vi "Pod Health Status Simulator.vi"(10 "Simulated Telemetry":T1={"Friction Brake (mA)"=300.0, "Mag Brake (mA)"=306.4516129032258, "Prim. Batt. (V)"=11.822168912654636, "Backup Batt. (V)"=11.62716511535498, "High Pressure (PSI)"=2438.59649122807, "Med. Pressure (PSI)"=254.3859649122807, "Low Pressure (PSI)"=50.29239766081871, "Brake Pressure (PSI)"=0.0, "ToF 1 (mm)"=10.75916230366492, "ToF 2 (mm)"=9.81675392670157, "ToF 3 (mm)"=10.44502617801047, "ToF 4 (mm)"=10.75916230366492, "Maglock 1 (mm)"=1.4705882352941175, "Maglock 2 (mm)"=1.1764705882352942, "Maglock 3 (mm)"=1.5294117647058822, "Maglock 4 (mm)"=1.2941176470588236} {"Brake Pressure (PSI)" scale=0.0..1000.0; "Maglock 4 (mm)" scale=0.0..15.0; "Maglock 3 (mm)" scale=0.0..15.0; "Maglock 2 (mm)" scale=0.0..15.0; "Maglock 1 (mm)" scale=0.0..15.0; "ToF 4 (mm)" scale=0.0..100.0; "ToF 3 (mm)" scale=0.0..100.0; "ToF 2 (mm)" scale=0.0..100.0; "ToF 1 (mm)" scale=0.0..100.0; "Low Pressure (PSI)" scale=0.0..1000.0; "Med. Pressure (PSI)" scale=0.0..1000.0; "High Pressure (PSI)" scale=0.0..1000.0; "Backup Batt. (V)" scale=0.0..15.0; "Prim. Batt. (V)" scale=0.0..15.0; "Mag Brake (mA)" scale=0.0..500.0; "Friction Brake (mA)" scale=0.0..500.0}, 11 "Pod Health Configuration":T2={"Power"={"Brake Max (mA)"=400.0, "Brake Min (mA)"=200.0, "Batt. Min (V)"=11.5, "Batt. Max (V)"=13.0}, "Pressure"={"HP Max (PSI)"=3000.0, "HP Min (PSI)"=2000.0, "MP Max (PSI)"=350.0, "MP Min (PSI)"=250.0, "LP Max (PSI)"=55.0, "LP Min (PSI)"=45.0, "BP Max (PSI)"=250.0, "BP Min (PSI)"=150.0}, "Position"={"Maglock Max (mm)"=3.0, "Maglock Min (mm)"=1.0, "Lev. Min (mm)"=30.0, "Lev. Max (mm)"=256.0}}) -> (2 "Pod Health":T3)   [LabVIEW 2014]
uses:
  Type Defs/PodHealth.ctl
  Type Defs/PodHealthConfig.ctl
  Type Defs/Telemetry.ctl
panel:
  in  "Reset 2":bool
  in  "Reset":bool
  in  "stop":bool
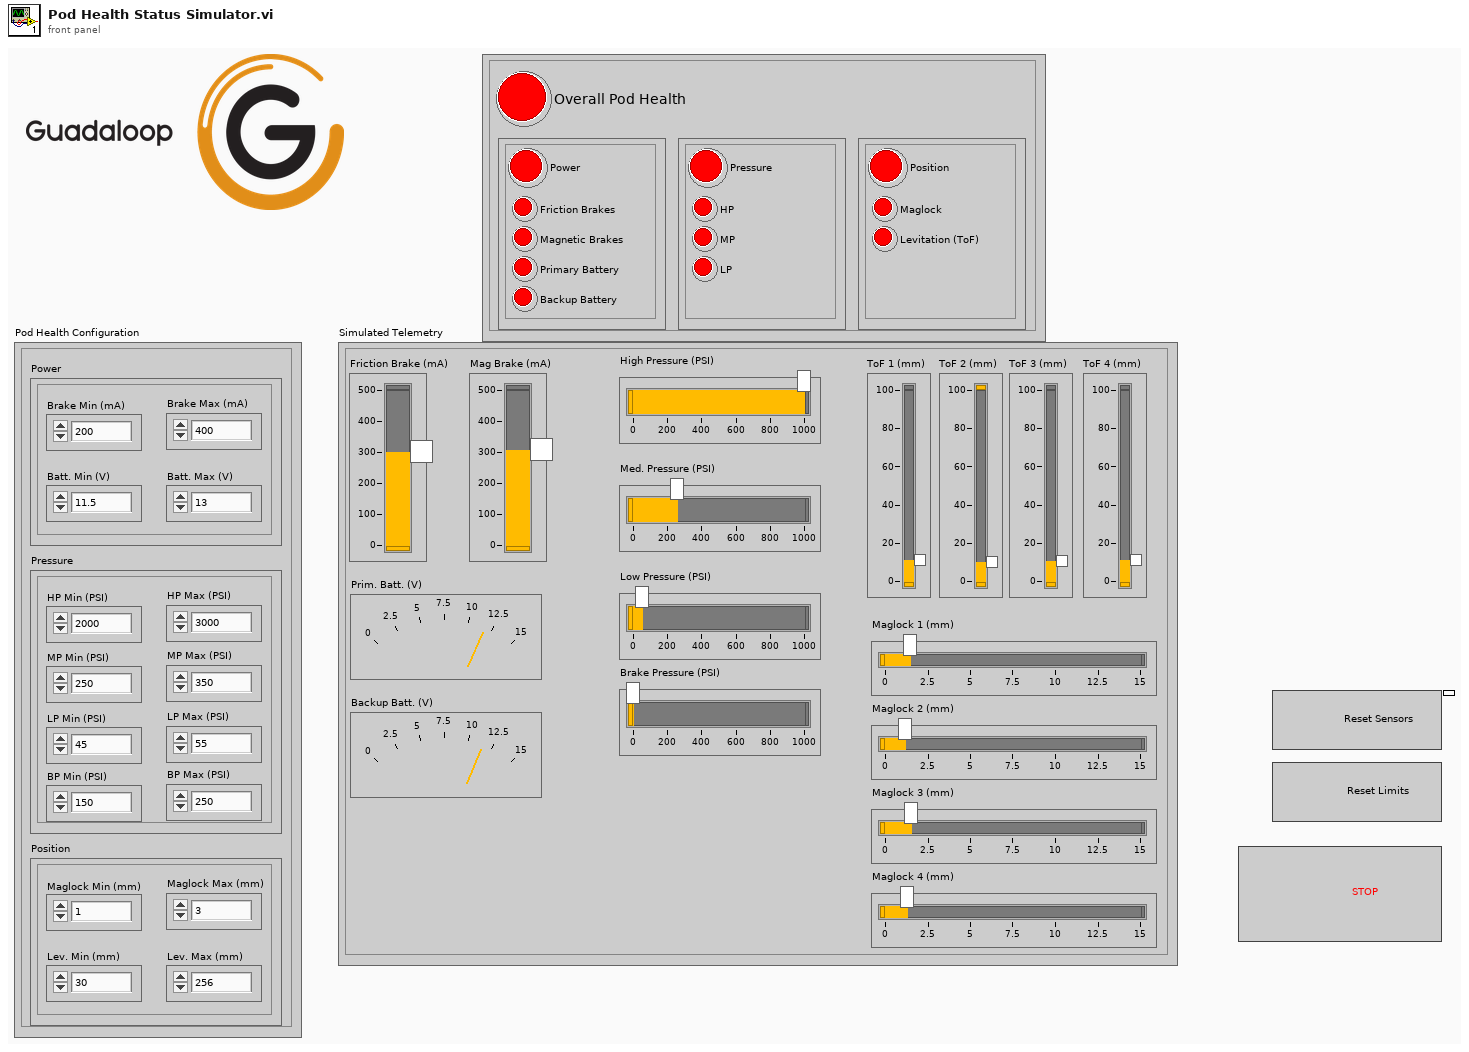
[diagram p1: front panel]
types:
  T1 = typedef "Telemetry.ctl" = cluster{"Friction Brake (mA)":dbl, "Mag Brake (mA)":dbl, "Prim. Batt. (V)":dbl, "Backup Batt. (V)":dbl, "High Pressure (PSI)":dbl, "Med. Pressure (PSI)":dbl, "Low Pressure (PSI)":dbl, "Brake Pressure (PSI)":dbl, "ToF 1 (mm)":dbl, "ToF 2 (mm)":dbl, "ToF 3 (mm)":dbl, "ToF 4 (mm)":dbl, "Maglock 1 (mm)":dbl, "Maglock 2 (mm)":dbl, "Maglock 3 (mm)":dbl, "Maglock 4 (mm)":dbl}
  T2 = typedef "PodHealthConfig.ctl" = cluster{"Power":cluster{"Brake Max (mA)":dbl, "Brake Min (mA)":dbl, "Batt. Min (V)":dbl, "Batt. Max (V)":dbl}, "Pressure":cluster{"HP Max (PSI)":dbl, "HP Min (PSI)":dbl, "MP Max (PSI)":dbl, "MP Min (PSI)":dbl, "LP Max (PSI)":dbl, "LP Min (PSI)":dbl, "BP Max (PSI)":dbl, "BP Min (PSI)":dbl}, "Position":cluster{"Maglock Max (mm)":dbl, "Maglock Min (mm)":dbl, "Lev. Min (mm)":dbl, "Lev. Max (mm)":dbl}}
  T3 = typedef "PodHealth.ctl" = cluster{"Overall Pod Health":bool, "Power":cluster{"Power":bool, "Friction Brakes":bool, "Magnetic Brakes":bool, "Primary Battery":bool, "Backup Battery":bool}, "Pressure":cluster{"Pressure":bool, "HP":bool, "MP ":bool, "LP":bool}, "Position":cluster{"Position":bool, "Maglock":bool, "Levitation (ToF)":bool}}
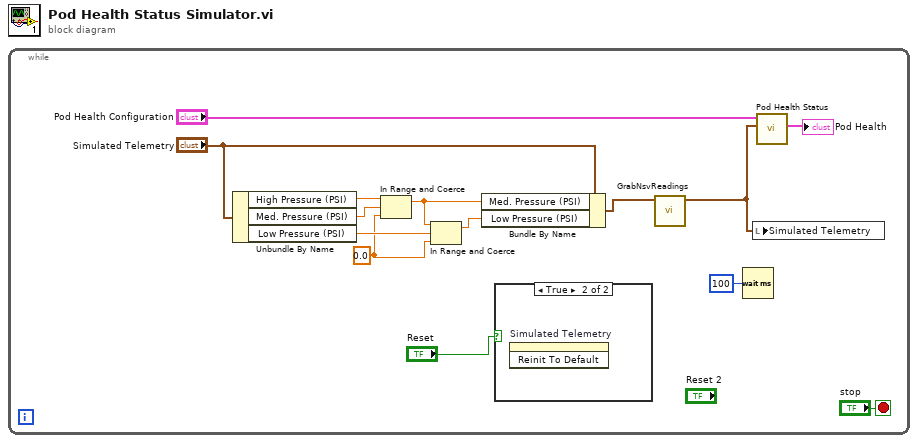
[diagram p0: block diagram]
diagram:
  n1 = while {
    stop <- "stop" stop-if-true
    w5 = 0.0 ("lower limit")
    n2 = Unbundle By Name("Simulated Telemetry") -> ("High Pressure (PSI)"=w11:dbl, "Med. Pressure (PSI)"=w10:dbl, "Low Pressure (PSI)"=w9:dbl)
    n3 = In Range and Coerce(upper limit=w11, x=w10, lower limit=w5) -> (coerced(x)=w8:dbl)  [unwired: 1 out]
    n4 = In Range and Coerce(upper limit=w8, x=w9, lower limit=w5) -> (coerced(x)=w7:dbl)  [unwired: 1 out]
    n5 = Bundle By Name(cluster="Simulated Telemetry", "Med. Pressure (PSI)"=w8, "Low Pressure (PSI)"=w7) -> (w1:T1)
    n6 = case shown="True" "Reset" {
      frame False {
      }
      frame True {
        n7 = invoke on="Simulated Telemetry" class="Clust (strict)" method="Reinit To Default"() -> ()  [unwired: 3 in, 3 out]
      }
    }
    n8 = call "GrabNsvReadings.vi"("Simulated Telemetry in"=w1) -> ("Simulated Telemetry out"=w2:T1)  [unwired: 10 in]
    n9 = Wait (ms)(milliseconds to wait=u32 100) -> ()  [unwired: 1 out]
    n10 = local write "Simulated Telemetry"(w2) -> ()
    n11 = call "Pod Health Status.vi"("Telemetry"=w2, "Pod Health Configuration"="Pod Health Configuration") -> ("Pod Health"=→"Pod Health":T3)  [unwired: 9 in]
  }
